vi "Transfer Images Data to UI.vi"(0 "fpga interface in":refnum<k20>, 1 "'stop' notifier":refnum<notifier>, 2 "Auto Vision Config":T1, 3 "measure call context in":refnum<class "Measure Call Context.lvclass">, 5 "Active Channel":string[](array[string]), 7 "number":i32, 11 "error in":errorcluster, 12 "References":T6, 13 "raw display notifier":refnum<notifier>) -> (4 "fpga interface out":refnum<k20>, 15 "error out":errorcluster)   [LabVIEW 2025, in "Automotive Vision.lvclass"]
doc: "Handles frame grabbing, and prepare data for sendig it to the UI."
uses:
  Automotive Vision.lvclass
  <vilib>/Plug-In SDKs/Measurements/Measure Call Context/Measure Call Context.lvclass
  <vilib>/rvi/interface/nirviReadWriteControl/nirviReadWriteControl.xnode
  ttashjia/GSE/Host/Common/GettingStarted_Common_148X_Host.lvlib
  ttashjia/GSE/Host/Common/Types/148x_Common_FPGA_Reference.ctl
  <instrlib>/FlexRIO/CSI-2/v2/Common/Types/LLP Data Type.ctl
  <instrlib>/FlexRIO/CSI-2/v2/Common/NI CSI-2 API Common v2.lvlib
  Automotive-Vision OOB Data Transfer/Automotive-Vision OOB Data Transfer.lvlib
  Measurement Results.ctl
  <resource>/objmgr/niflexrioapiChannel.rc
  <instrlib>/FlexRIO/API/Host/v1/NI FlexRIO API v1.lvlib
  <instrlib>/FlexRIO/API/Host/v1/NI FlexRIO/API/Get Property Reference - Fpga Small.vi
  NiFpgaLv.dll
  <vilib>/Utility/error.llb/Error Cluster From Error Code.vi
  <vilib>/rvi/interface/Simulation/niFpgaSimulationCallBeginRW.vi
  <vilib>/rvi/errors/niLvFpgaAdjustHostInterfaceError.vi
  <vilib>/vision/Image Controls.llb/IMAQ Image.ctl
  ttashjia/GSE/Host/Common/Types/RAW Interpretation for Display.ctl
  ttashjia/GSE/Host/Common/Types/Serial Channel Display Parameters.ctl
  embedded data item.ctl
  embedded data.ctl
  register.ctl
  autovision_config.ctl
panel:
  out "output cluster 2":T5={"ACQ. IN PROGRESS"=FALSE, "IMAGE PIXEL DATA"=[], "ACQ. DURATION (s)"=0.0, "SOURCE RATE (fps)"=0.0, "BYTES ACQUIRED"=0, "FRAME COUNT"=0, "POC VOLTAGE (V)"=0.0, "POC CURRENT (A)"=0.0, "ERROR"=FALSE, "STATE MESSAGE"="Initializing...", "IMAGE DATA"="", "OOB gRPC Port"=0, "HEIGHT"=0, "WIDTH"=0, "FRAME COUNT BYTES"=[], "REGISTERS"=[], "COUNT LENGTH"=0} {"BYTES ACQUIRED" format="%#.6p"}
  in  "output cluster":T5={"ACQ. IN PROGRESS"=FALSE, "IMAGE PIXEL DATA"=[], "ACQ. DURATION (s)"=0.0, "SOURCE RATE (fps)"=0.0, "BYTES ACQUIRED"=0, "FRAME COUNT"=0, "POC VOLTAGE (V)"=0.0, "POC CURRENT (A)"=0.0, "ERROR"=FALSE, "STATE MESSAGE"="Initializing...", "IMAGE DATA"="", "OOB gRPC Port"=0, "HEIGHT"=0, "WIDTH"=0, "FRAME COUNT BYTES"=[], "REGISTERS"=[], "COUNT LENGTH"=0} {"BYTES ACQUIRED" format="%#.6p"}
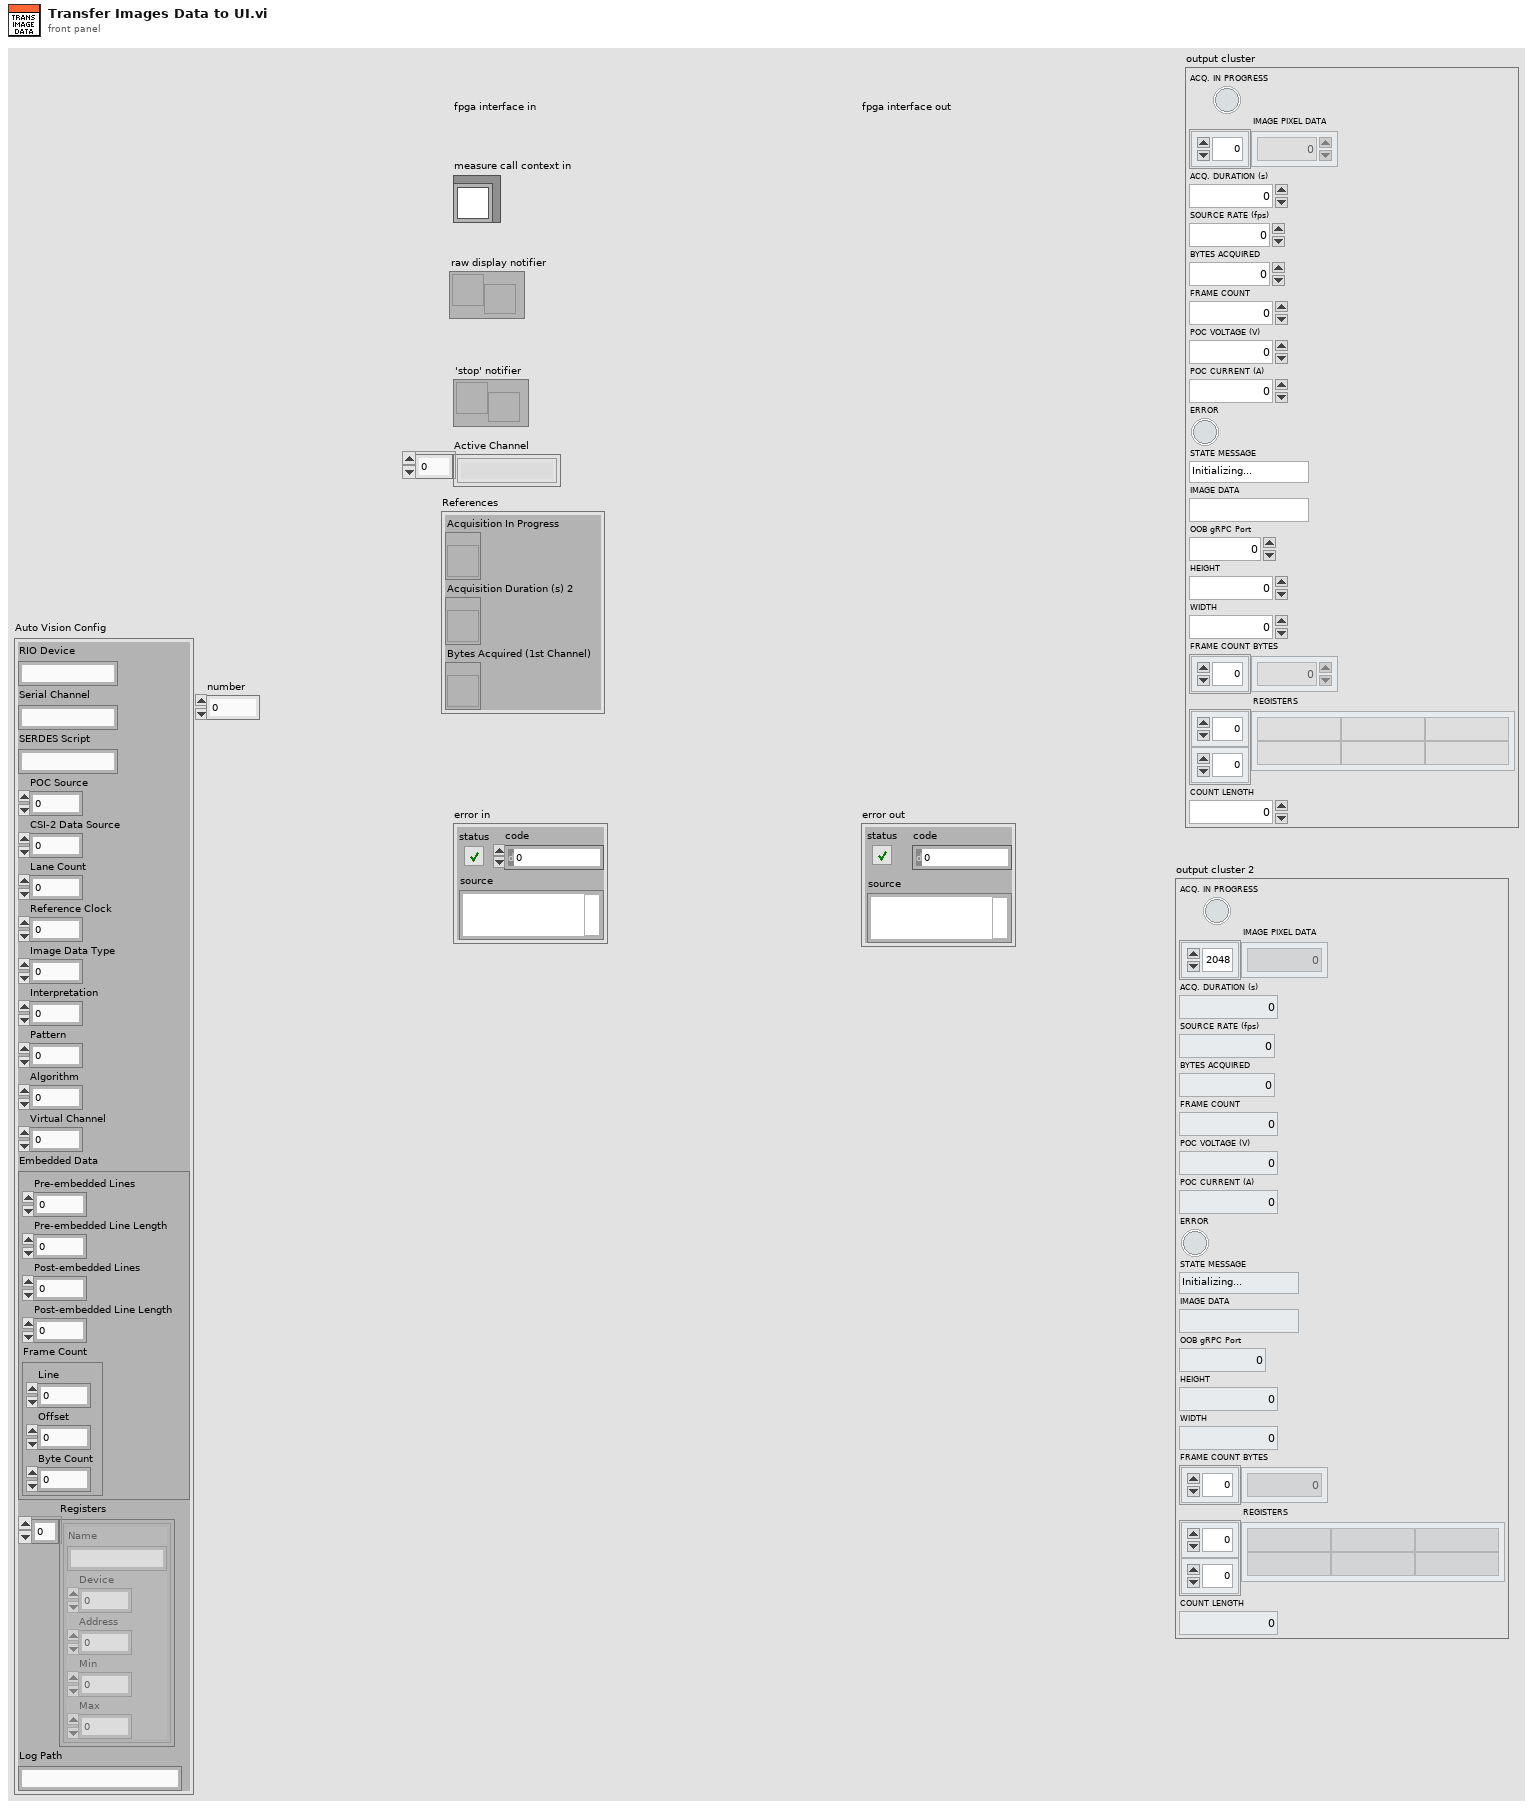
[diagram p1: front panel]
types:
  T1 = typedef "Automotive Vision.lvclass/autovision_config.ctl" = cluster{"RIO Device":string, "Serial Channel":string, "SERDES Script":string, "POC Source":u32, "CSI-2 Data Source":u32, "Lane Count":u32, "Reference Clock":dbl, "Image Data Type":u32, "Interpretation":u32, "Pattern":u32, "Algorithm":u32, "Virtual Channel":u32, "Embedded Data":T2, "Registers":T4[], "Log Path":string}
  T2 = typedef "Automotive Vision.lvclass/embedded data.ctl" = cluster{"Pre-embedded Lines":dbl, "Pre-embedded Line Length":dbl, "Post-embedded Lines":dbl, "Post-embedded Line Length":dbl, "Frame Count":T3}
  T3 = typedef "Automotive Vision.lvclass/embedded data item.ctl" = cluster{"Line":dbl, "Offset":dbl, "Byte Count":dbl}
  T4 = typedef "Automotive Vision.lvclass/register.ctl" = cluster{"Name":string, "Device":u8, "Address":u16, "Min":u16, "Max":u16}
  T5 = typedef "Automotive Vision.lvclass/Measurement Results.ctl" = cluster{"ACQ. IN PROGRESS":bool, "IMAGE PIXEL DATA":u32[], "ACQ. DURATION (s)":dbl, "SOURCE RATE (fps)":dbl, "BYTES ACQUIRED":u64, "FRAME COUNT":u64, "POC VOLTAGE (V)":dbl, "POC CURRENT (A)":dbl, "ERROR":bool, "STATE MESSAGE":string, "IMAGE DATA":string, "OOB gRPC Port":i32, "HEIGHT":u64, "WIDTH":u64, "FRAME COUNT BYTES":u32[], "REGISTERS":string[][], "COUNT LENGTH":u64}
  T6 = cluster{"Acquisition In Progress":refnum<vi>, "Acquisition Duration (s) 2":refnum<vi>, "Bytes Acquired (1st Channel)":refnum<vi>}
  T7 = typedef "NI CSI-2 API Common v2.lvlib/LLP Data Type.ctl" = enum8{"Frame Start", "Frame End", "Line Start", "Line End", "End of Transmission", "Reserved 0", "Reserved 1", "Reserved 2", "Generic Short Packet 1", "Generic Short Packet 2", "Generic Short Packet 3", "Generic Short Packet 4", "Generic Short Packet 5", "Generic Short Packet 6", "Generic Short Packet 7", "Generic Short Packet 8", "Null", "Blanking Data", "Embedded 8-bit non Image Data", "Generic Long Packet 1", "Generic Long Packet 2", "Generic Long Packet 3", "Generic Long Packet 4", "Reserved 3", "YUV420 8-bit", "YUV420 10-bit", "Legacy YUV420 8-bit", "Reserved 4", "YUV420 8-bit Chroma Shifted", "YUV420 10-bit Chroma Shifted", "YUV422 8-bit", "YUV422 10-bit", "RGB444", "RGB555", "RGB565", "RGB666", "RGB888", "Reserved 5", "Reserved 6", "RAW 24", "RAW 6", "RAW 7", "RAW 8", "RAW 10", "RAW 12", "RAW 14", "RAW 16", "RAW 20", "User Defined 8-bit Data 1", "User Defined 8-bit Data 2", "User Defined 8-bit Data 3", "User Defined 8-bit Data 4", "User Defined 8-bit Data 5", "User Defined 8-bit Data 6", "User Defined 8-bit Data 7", "User Defined 8-bit Data 8", "USL Command", "Reserved 7", "Reserved 8", "Reserved 9", "Reserved 10", "Reserved 11", "Reserved 12", "LRTE EPD Spacer"}
  T8 = cluster{"serial channel":fxp<+,3,3>, "frame number":u16, "data type":T7, "width":u16, "height":u16, "image bytes":u32, "total bytes":u32, "little endian":bool, "Status":string}
  T9 = typedef "GettingStarted_Common_148X_Host.lvlib/148x_Common_FPGA_Reference.ctl" = refnum<k20>
  T10 = typedef "Automotive-Vision OOB Data Transfer.lvlib/OOB to Logic Data.ctl" = cluster{"PauseResume":bool, "ExportPath":string, "ExportType":u16, "Export":bool}
  T11 = typedef "GettingStarted_Common_148X_Host.lvlib/Serial Channel Display Parameters.ctl" = cluster{"images":cluster{"grayscale":T12, "color":T12}, "RAW parameters":cluster{"interpretation":T13, "bayer parameters":cluster{"pattern":i32, "algorithm":i32, "red gain":dbl, "green gain":dbl, "blue gain":dbl}}}
  T12 = typedef "IMAQ Image.ctl" = refnum<image>
  T13 = typedef "GettingStarted_Common_148X_Host.lvlib/RAW Interpretation for Display.ctl" = enum16{"Grayscale", "Bayer", "RGB", "YUV422", "YUV420", "Legacy YUV420"}
  T14 = typedef "GettingStarted_Common_148X_FPGA.lvlib/Image Metadata.ctl" = cluster{"serial channel":fxp<+,3,3>, "frame number":u16, "data type":T7, "width":u16, "height":u16, "image bytes":u32, "total bytes":u32, "little endian":bool}
  T15 = cluster{"image pixel data fifo overflow":bool, "image metadata fifo overflow":bool}[]
  T16 = cluster{"image pixel data fifo overflow":bool, "image metadata fifo overflow":bool}
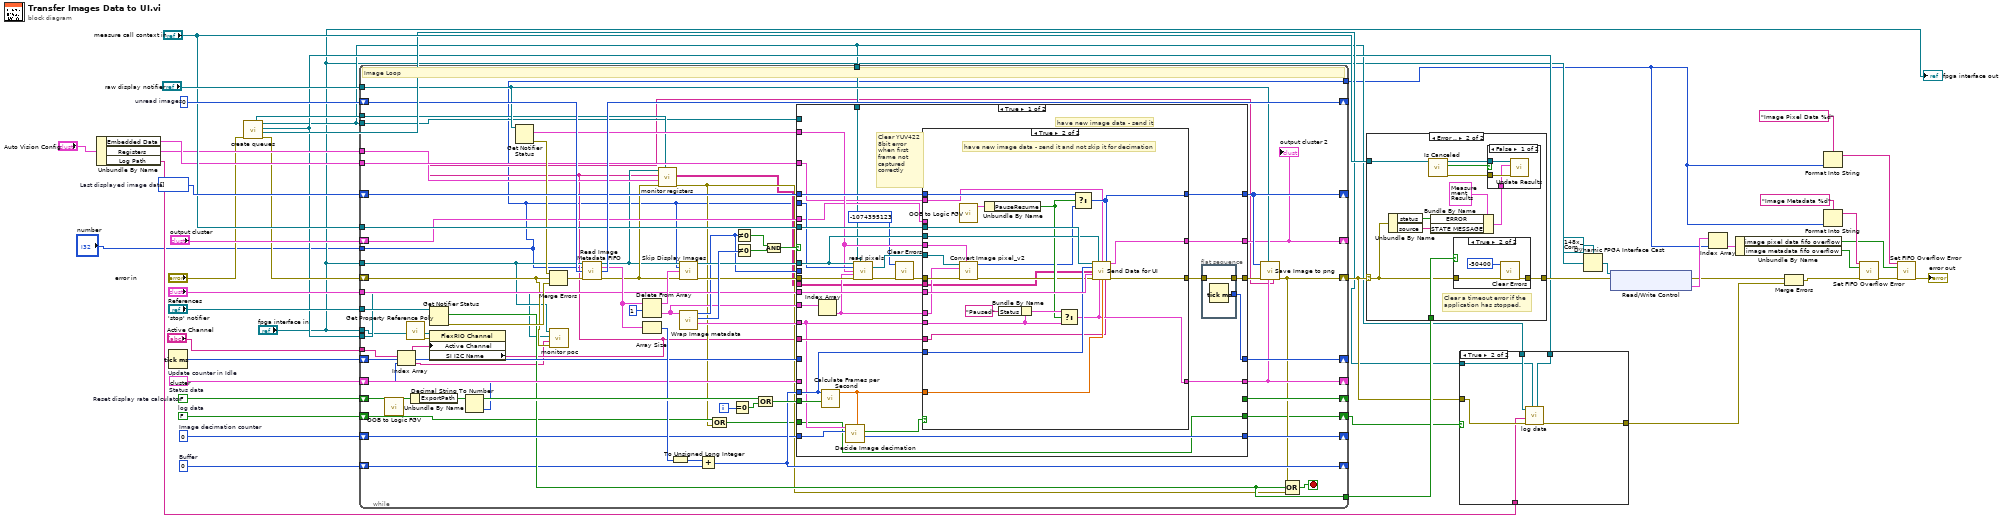
[diagram p0: block diagram]
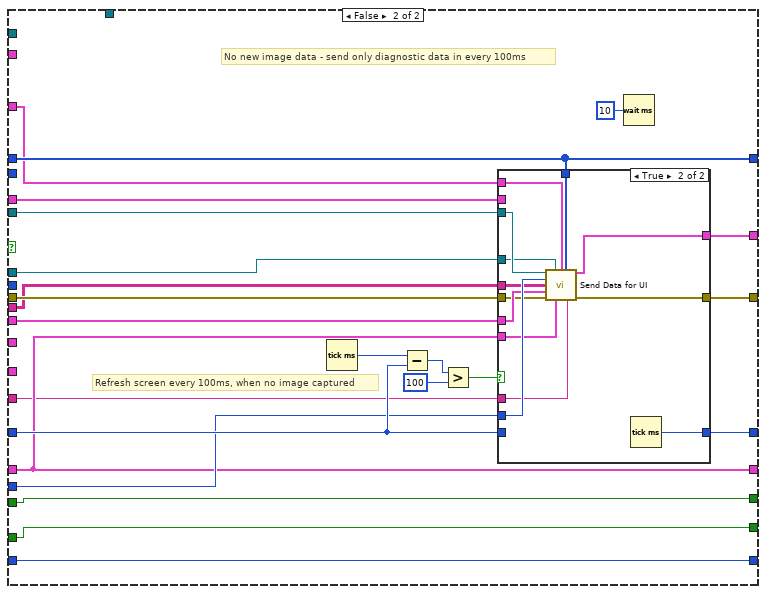
[diagram p4: hidden frame]
diagram:
  w14 = FALSE  # log data
  w24 = T8 {"serial channel"=0.0, "frame number"=0, "data type"=enum."Frame Start", "width"=0, "height"=0, "image bytes"=0, "total bytes"=0, "little endian"=FALSE, "Status"="Ready for Acquisition"}  # Status data
  w26 = u32 0  # Image decimation counter
  w27 = u32[] []  # Last displayed image data
  w31 = u32 0  # Buffer
  w32 = FALSE  # Reset display rate calculator
  w46 = u32 0  # unread images
  n1 = Unbundle By Name("Auto Vision Config") -> ("Embedded Data"=w19:T2, "Registers"=w18:T4[], "Log Path"=w8:string)
  n2 = Tick Count (ms) "Update counter in Idle"() -> (millisecond timer value=w28:u32)
  n3 = call "create queues.vi"("error in (no error)"="error in") -> ("error out"=w16:errorcluster, "i2c queue out"=w7:refnum<queue>, "power monitor queue out"=w6:refnum<queue>, "image queue out"=w5:refnum<queue>, "register monitor queue out"=w15:refnum<queue>)  [unwired: 6 in]
  n4 = while {
    shift-right: [w78] -> w10
    shift-left: w16 -> [w60]
    tunnel: "fpga interface in" -> [w59]
    shift-right: [w114] -> _
    shift-left: w46 -> [w105]
    shift-right: [w109] -> _
    shift-left: w32 -> [w106]
    shift-right: [w98] -> _
    shift-left: w31 -> [w82]
    tunnel: [w84] -> w30
    tunnel: "'stop' notifier" -> [w96]
    shift-right: [w93] -> _
    shift-left: w28 -> [w94]
    shift-right: [w81] -> _
    shift-left: w27 -> [w92]
    shift-right: [w90] -> _
    shift-left: w26 -> [w91]
    tunnel: "References" -> [w89]
    tunnel: "measure call context in" -> [w88]
    shift-right: [w79] -> _
    shift-left: w24 -> [w87]
    tunnel: "raw display notifier" -> [w77]
    tunnel: w19 -> [w73]
    shift-right: [w71] -> _
    shift-left: "output cluster" -> [w72]
    tunnel: w18 -> [w69]
    tunnel: w15 -> [w67]
    shift-right: [w61] -> w13
    shift-left: w14 -> [w66]
    tunnel: w5 -> [w63]
    tunnel: w6 -> [w58]
    tunnel: w5 -> [w57]
    tunnel: "fpga interface in" -> [w52]
    tunnel: "Active Channel" -> [w51]
    tunnel: [w47] -> w2
    tunnel: "number" -> [w47]
    i -> [w113]
    stop <- w115 stop-if-true
    # "Image Loop"
    n5 = call "OOB to Logic FGV.vi"() -> ("OOB to Logic Data out"=w56:T10)  [unwired: 10 in, 1 out]
    n6 = call-poly <instrlib>:"Get Property Reference Poly.vi"("fpga interface in"=w52) -> ("error out"=w53:errorcluster, "property reference"=w54:refnum<k20>)  [unwired: 5 in, 1 out]
    n7 = Unbundle By Name(w56) -> ("ExportPath"=w55:string)
    n8 = Get Notifier Status(notifier=w96) -> (current notification=w84:bool, error out=w116:errorcluster)  [unwired: 1 in, 3 out]
    n9 = Decimal String To Number(string=w55) -> (number=w48:i32)  [unwired: 2 in, 1 out]
    n10 = Index Array(array=w51, index=w48) -> (element=w49:string)
    n11 = property class="FlexRIO Channel"(reference=w54, error in=w53, "Active Channel"=w49) -> ("SI I2C Name"=w50:string)  [unwired: 2 out]
    n12 = Get Notifier Status(notifier=w77) -> (current notification=w75:T11[], error out=w76:errorcluster)  [unwired: 1 in, 3 out]
    n13 = Merge Errors(w76, w60, w116) -> (w95:errorcluster)
    n14 = call "monitor poc.vi"("error in"=w60, "Active Channel"=w49, "power monitor queue in"=w58, "fpga interface in"=w59) -> ()  [unwired: 7 in, 1 out]
    n15 = call "Read Image Metadata FIFO.vi"("fpga inteface in"=w59, "display channel number"=w47, "number of images"=w105, "error in (no error)"=w95) -> ("fpga interface out"=w68:refnum<k20>, "image metadata"=w97:T14[], "images remaining"=w114:u32, "error out"=w70:errorcluster)  [unwired: 8 in]
    n16 = Delete From Array(array=w97, length=1) -> (deleted portion=w74:T14[], array with subset deleted=w100:T14[])  [unwired: 1 in]
    n17 = Array Size(array=w97) -> (size(s)=w99:i32)
    n18 = call "monitor registers.vi"("register monitor queue"=w67, "error in"=w70, "Registers"=w69, "bus instance name"=w50, "fpga interface in"=w68) -> ("error out"=w65:errorcluster, "registers out"=w62:string[][])  [unwired: 3 in, 2 out]
    n19 = To Unsigned Long Integer(number=w99) -> (unsigned 32bit integer=w83:u32)
    n20 = call "Skip Display Images.vi"("fpga interface in"=w68, "display channel number"=w47, "image metadata"=w100, "error in (no error)"=w70) -> ("fpga interface out"=w102:refnum<k20>, "error out"=w101:errorcluster)  [unwired: 10 in]
    n21 = call "Wrap Image metadata.vi"("image metadata"=w74) -> ("element"=w86:T8, "Numeric"=w104:i32, "total bytes"=w85:u32)  [unwired: 8 in]
    n22 = Add(x=w83, y=w82) -> (x+y=w98:u32)
    n23 = Compound Arithmetic op=OR(w66, w65) -> (w64:bool)
    n24 = Equal To 0?(x=w113) -> (x = 0?=w107:bool)
    n25 = Not Equal To 0?(x=w85) -> (x != 0?=w111:bool)
    n26 = Not Equal To 0?(x=w104) -> (x != 0?=w112:bool)
    n27 = Compound Arithmetic op=OR(w106, w107) -> (w108:bool)
    n28 = Compound Arithmetic op=AND(w111, w112) -> (w110:bool)
    n29 = case shown="True" w110 {
      tunnel: w101 -> [w134 w186]
      tunnel: w102 -> [w133 w184]
      tunnel: w47 -> [w132 _]
      tunnel: [w146 w193] -> w80
      tunnel: w108 -> [w137 w200]
      tunnel: [_ w200] -> w109
      tunnel: w98 -> [w143 w190]
      tunnel: w85 -> [_ _]
      tunnel: w86 -> [w127 _]
      tunnel: w88 -> [w148 w187]
      tunnel: w89 -> [w147 w201]
      tunnel: w94 -> [_ w192]
      tunnel: [w145 w194] -> w93
      tunnel: w92 -> [w142 w191]
      tunnel: [w144 w191] -> w81
      tunnel: w91 -> [w141 w189]
      tunnel: [w140 w189] -> w90
      tunnel: w87 -> [_ w188]
      tunnel: [w138 w188] -> w79
      tunnel: w50 -> [w136 w185]
      tunnel: w75 -> [w128 _]
      tunnel: w74 -> [w131 _]
      tunnel: w73 -> [w122 w183]
      tunnel: w72 -> [w120 w181]
      tunnel: [w121 w182] -> w71
      tunnel: w64 -> [w118 w179]
      tunnel: w63 -> [_ _]
      tunnel: w62 -> [w119 w180]
      tunnel: [w118 w179] -> w61
      tunnel: w57 -> [w117 _]
      frame True {
        # "Clear YUV422 8bit error when first frame not captured correctly"
        # "have new image data - send it"
        n30 = Index Array(array=w131) -> (element=w130:T14)  [unwired: 1 in]
        n31 = call <vilib>:"Calculate Frames per Second.vi"("Reset"=w137, "Buffer Number"=w143) -> ("Acquired Frames/s"=w126:dbl)  [unwired: 7 in, 2 out]
        n32 = call "Decide Image decimation.vi"("FPS"=w126, "Image decimation counter in"=w141, "element in"=w127) -> ("Image decimation counter out"=w140:u32, "send current image data"=w139:bool)  [unwired: 7 in]
        n33 = call "read pixels.vi"("fpga interface in"=w133, "image queue in"=w117, "display channel number"=w132, "serial channel display parameters"=w128, "image metadata"=w130, "error in (no error)"=w134) -> ("display image"=w129:T12, "error out"=w124:errorcluster)  [unwired: 7 in, 1 out]
        n34 = call <vilib>:"Clear Errors.vi"("error in (no error)"=w124, "specific error code to clear (0: all)"=-1074395123) -> ("error out"=w123:errorcluster)  [unwired: 4 in, 1 out]
        n35 = case shown="True" w139 {
          tunnel: [w150 w168] -> w135
          tunnel: w126 -> [_ w176]
          tunnel: w127 -> [w151 w163]
          tunnel: w148 -> [_ w175]
          tunnel: w147 -> [_ w174]
          tunnel: [w152 w173] -> w144
          tunnel: w143 -> [_ w172]
          tunnel: w142 -> [w152 w171]
          tunnel: [w151 w170] -> w138
          tunnel: w133 -> [_ w169]
          tunnel: w136 -> [_ w162]
          tunnel: w123 -> [w150 w161]
          tunnel: w129 -> [_ w159]
          tunnel: w130 -> [_ w157]
          tunnel: w128 -> [_ w156]
          tunnel: w122 -> [_ w155]
          tunnel: [w149 w154] -> w121
          tunnel: w120 -> [w149 _]
          tunnel: w119 -> [_ w153]
          frame False {
            # "have new image data - but skip the sending to not overload UI with data transfer"
          }
          frame True {
            # "have new image data - send it and not skip it for decimation"
            n36 = call "OOB to Logic FGV.vi"() -> ("OOB to Logic Data out"=w165:T10)  [unwired: 10 in, 1 out]
            n37 = call "Convert Image pixel_v2.vi"("serial channel display parameters"=w156, "error in"=w161, "image metadata"=w157, "Refnum in"=w159) -> ("error out"=w160:errorcluster, "Image Pixels (U32)"=w158:u32[])  [unwired: 6 in]
            n38 = Unbundle By Name(w165) -> ("PauseResume"=w164:bool)
            n39 = Bundle By Name(cluster=w163, "Status"="Paused") -> (w167:T8)
            n40 = Select(t=w167, s=w164, f=w163) -> (s? t:f=w170:T8)
            n41 = Select(t=w171, s=w164, f=w158) -> (s? t:f=w173:u32[])
            n42 = call "Send Data for UI.vi"("Measure Call Context in"=w175, "fpga interface in"=w169, "Embedded Data"=w155, "Last displayed image data"=w173, "FrameCount"=w172, "registers"=w153, "References"=w174, "error in"=w160, "Status data"=w170, "SOURCE RATE (fps)"=w176, "Active Channel"=w162) -> ("output cluster"=w154:T5, "error out"=w168:errorcluster)  [unwired: 3 in]
          }
        }
        n43 = flat-sequence {
          tunnel: [w178] -> w146
          tunnel: w135 -> [w178]
          tunnel: [w177] -> w145
          frame #0 {
            n44 = Tick Count (ms)() -> (millisecond timer value=w177:u32)
          }
        }
      }
      frame False {
        # "Refresh screen every 100ms, when no image captured"
        # "No new image data - send only diagnostic data in every 100ms"
        n45 = Tick Count (ms)() -> (millisecond timer value=w198:u32)
        n46 = Subtract(x=w198, y=w192) -> (x-y=w197:u32)
        n47 = Greater?(x=w197, y=u32 100) -> (0:w195:bool)
        n48 = case shown="True" w195 {
          tunnel: w186 -> [w204 w210]
          tunnel: [w204 w217] -> w193
          tunnel: w188 -> [_ w212]
          tunnel: w201 -> [_ w213]
          tunnel: [w203 w216] -> w194
          tunnel: w192 -> [w203 _]
          tunnel: w191 -> [_ w215]
          tunnel: w190 -> [_ w214]
          tunnel: w187 -> [_ w211]
          tunnel: w185 -> [_ w209]
          tunnel: w184 -> [_ w208]
          tunnel: w183 -> [_ w207]
          tunnel: [w202 w206] -> w182
          tunnel: w181 -> [w202 _]
          tunnel: w180 -> [_ w205]
          frame False {
          }
          frame True {
            n49 = call "Send Data for UI.vi"("Measure Call Context in"=w211, "fpga interface in"=w208, "Embedded Data"=w207, "Last displayed image data"=w215, "FrameCount"=w214, "registers"=w205, "References"=w213, "error in"=w210, "Status data"=w212, "Active Channel"=w209) -> ("output cluster"=w206:T5, "error out"=w217:errorcluster)  [unwired: 4 in]
            n50 = Tick Count (ms)() -> (millisecond timer value=w216:u32)
          }
        }
        n51 = Wait (ms)(milliseconds to wait=u32 10) -> ()  [unwired: 1 out]
      }
    }
    "output cluster 2" <- w71
    n52 = call "Save Image to png.vi"("Channel"=w50, "image metadata"=w79, "raw display notifier"=w77, "error in"=w80, "Last displayed image data"=w81) -> ("error out"=w78:errorcluster)  [unwired: 6 in]
    n53 = Compound Arithmetic op=OR(w78, w84, w65) -> (w115:bool)
  }
  n54 = case shown="Error .." w10 {
    selector: w10 -> [w218 w222]
    tunnel: [w218 w229] -> w41
    tunnel: w30 -> [_ w228]
    tunnel: "measure call context in" -> [_ w219]
    frame No Error {
    }
    frame Error {
      # "Clear a timeout error if the application has stopped."
      n55 = Unbundle By Name(w222) -> ("status"=w221:bool, "source"=w220:string)
      n56 = call <vilib>:"Is Canceled.vi"("measure call context in"=w219) -> ("error out"=w226:errorcluster, "is canceled?"=w225:bool, "measure call context out"=w227:refnum<class "Measure Call Context.lvclass">)  [unwired: 8 in]
      n57 = Bundle By Name(cluster=T5 {"ACQ. IN PROGRESS"=FALSE, "IMAGE PIXEL DATA"=[], "ACQ. DURATION (s)"=0.0, "SOURCE RATE (fps)"=0.0, "BYTES ACQUIRED"=0, "FRAME COUNT"=0, "POC VOLTAGE (V)"=0.0, "POC CURRENT (A)"=0.0, "ERROR"=FALSE, "STATE MESSAGE"="", "IMAGE DATA"="", "OOB gRPC Port"=0, "HEIGHT"=0, "WIDTH"=0, "FRAME COUNT BYTES"=[], "REGISTERS"=[], "COUNT LENGTH"=0} ("Measurement Results"), "ERROR"=w221, "STATE MESSAGE"=w220) -> (w223:T5)
      n58 = case shown="True" w228 {
        tunnel: w222 -> [w233 w236]
        tunnel: [w233 w234] -> w229
        frame False {
        }
        frame True {
          n59 = call <vilib>:"Clear Errors.vi"("error in (no error)"=w236, "specific error code to clear (0: all)"=-50400 ("y")) -> ("error out"=w234:errorcluster)  [unwired: 4 in, 1 out]
        }
      }
      n60 = case shown="False" w225 {
        tunnel: w227 -> [w232 _]
        tunnel: w226 -> [w231 _]
        tunnel: w223 -> [w230 _]
        frame False {
          n61 = call <vilib>:"Update Results.vi"("error in"=w231, "measurement results"=w230, "measure call context in"=w232) -> ()  [unwired: 7 in, 2 out]
        }
        frame True {
        }
      }
    }
  }
  n62 = case shown="True" w13 {
    tunnel: w10 -> [w237 w243]
    tunnel: [w237 w242] -> w9
    tunnel: w8 -> [_ w241]
    tunnel: w6 -> [_ w240]
    tunnel: w5 -> [_ w239]
    tunnel: w7 -> [_ w238]
    frame False {
    }
    frame True {
      n63 = call "log data.vi"("power monitor queue in"=w240, "i2c queue in"=w238, "error in"=w243, "path"=w241, "image queue in"=w239) -> ("error out"=w242:errorcluster)  [unwired: 6 in]
    }
  }
  n64 = Dynamic FPGA Interface Cast(Session In=T9 refnum ("FPGA VI Reference Out"), Type="fpga interface in") -> (Session Out=w42:T9)
  n65 = xnode ("Read/Write Control")("FPGA VI Reference In"=w42, "error in"=w41) -> ("error out"=w12:errorcluster, "display channel status"=w44:T15)  [unwired: 1 out]
  n66 = Index Array(array=w44, index=w2) -> (element=w45:T16)
  n67 = Unbundle By Name(w45) -> ("image pixel data fifo overflow"=w34:bool, "image metadata fifo overflow"=w33:bool)
  n68 = Merge Errors(w12, w9) -> (w11:errorcluster)
  n69 = Format Into String(format string="Image Pixel Data %d", w2) -> (resulting string=w36:string)  [unwired: 2 in, 1 out]
  n70 = Format Into String(format string="Image Metadata %d", w2) -> (resulting string=w35:string)  [unwired: 2 in, 1 out]
  n71 = call "Set FIFO Overflow Error.vi"("fifo name"=w35, "overflow"=w33, "error in (no error)"=w11) -> ("error out"=w38:errorcluster)  [unwired: 12 in]
  n72 = call "Set FIFO Overflow Error.vi"("fifo name"=w36, "overflow"=w34, "error in (no error)"=w38) -> ("error out"=→"error out":errorcluster)  [unwired: 12 in]
  "fpga interface out" <- "fpga interface in"
